vi "EasyFitTransients.vi"(11 "InputData":T3(array[cluster])=[{"JV metrics"=[0.0, 0.004688074, 0.005002861, 0.0053417254, 0.0056762234, 0.0060026976, 0.006369476, 0.0066977106, 0.0070325956, 0.007371202, 0.007696711, 0.008035217, 0.008369455, 0.008697365, 0.0090301, 0.009363418, 0.009698967, 0.010032594, 0.010363362, 0.010703604, 0.01102955, 0.011368416, 0.011698721, 0.012031753, 0.012363813, 0.012696692, 0.013029694, 0.0133624505, 0.013696079, 0.014036833, 0.0143676335, 0.014702026, 0.015034515, 0.015362716, 0.01570068, 0.016029574, 0.016367266, 0.016696516, 0.017030975, 0.01736351, 0.017702773, 0.01802998, 0.018363293, 0.018697608, 0.019032346, 0.019362444, 0.019695722, 0.020032562, 0.0203697], "JV metrics"=[0.69321656, -3.15312e-05, -0.00017485018, -3.621295e-05, 6.4908316e-05, -2.1567195e-05, -2.285478e-05, -7.566182e-05, -0.00020427264, 4.1995507e-05, -0.00015639109, -0.00020229832, -0.00010161646, -0.0001144569, -0.00020186052, -0.00013796492, -0.00014203244, 8.4075975e-05, -2.4384806e-05, -7.140644e-05, 0.00012004285, -7.328456e-06, -0.00010339845, 0.0001509544, 4.349697e-05, 6.881247e-05, -0.0001570559, -3.9619877e-06, -0.00022902519, -4.6681085e-05, -0.0001399173, 7.6152726e-05, -0.0001232961, -0.00024506752, -0.00010704884, -0.00012851319, -0.00014125218, -7.473238e-07, 0.0001521912, -1.1394733e-05, -0.00019358074, 9.507881e-06, 1.6228494e-05, 5.089255e-05, 0.00014946784, 0.00020754292, -0.00022141216, -9.01446e-05, 5.6048953e-05]}]) -> ()   [LabVIEW 2020]
uses:
  <vilib>/Analysis/NI_AALPro.lvlib
panel:
  out "T80 (h)":dbl[](array[numeric])=[nan]
  in  "linear fit: parameter bounds":T1={"slope min"=-inf, "slope max"=inf, "intercept min"=-inf, "intercept max"=inf}
  in  "exponential fit parameter bounds":T2={"amp min"=-inf, "amp max"=inf, "damping min"=-inf, "damping max"=inf, "offset min"=0.0, "offset max"=0.0}
  out "Fitresults":dbl[][](array[numeric])=[[nan, nan, 0.0, nan]]
  out "Cursors":dbl[](array[numeric])=[0.7645161290322581, 5.903225806451613]
  in  "Exit Button":bool
  in  "Fit Button":bool
  in  "Fit function":bool
  out "AgingData":T3(graph)
  # "tau (h) / m (1/h)     A                     c             residue"
  # "from (h):"
  # "exponential\nAexp(dx)+c"
  # "linear\nmt +c"
  # "to (h):"
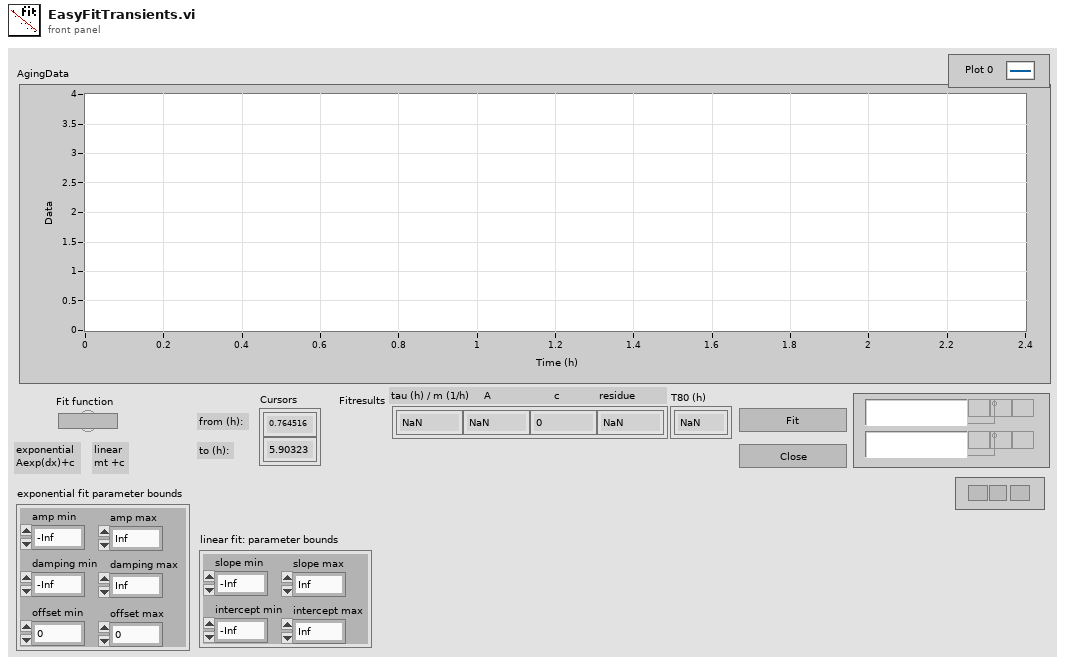
[diagram p1: front panel]
types:
  T1 = cluster{"slope min":dbl, "slope max":dbl, "intercept min":dbl, "intercept max":dbl}
  T2 = cluster{"amp min":dbl, "amp max":dbl, "damping min":dbl, "damping max":dbl, "offset min":dbl, "offset max":dbl}
  T3 = cluster{"JV metrics":sgl[], "JV metrics":sgl[]}[]
  T4 = typedef "LVCursorListTypeDef.ctl" = cluster{"Name":string, "Color":u32, "Style":u8, "Point Style":u8, "Name Visible":bool, "Allow Drag":bool, "Cursor Mode":u32, "Plot":i32, "Index":i32, "Position":cluster{"X":dbl, "Y":dbl}, "X Scale":u32, "Y Scale":u32, "Watch Plots":i32[], "Watch All Plots":bool, "Plot Area":i32, "Label Offset":cluster{"X":dbl, "Y":dbl}}[]
  T5 = cluster{"Name":string, "Color":u32, "Style":u8, "Point Style":u8, "Name Visible":bool, "Allow Drag":bool, "Cursor Mode":u32, "Plot":i32, "Index":i32, "Position":cluster{"X":dbl, "Y":dbl}, "X Scale":u32, "Y Scale":u32, "Watch Plots":i32[], "Watch All Plots":bool, "Plot Area":i32, "Label Offset":cluster{"X":dbl, "Y":dbl}}
  T6 = cluster{"JV metrics":sgl[], "Best Linear Fit":dbl[]}[]
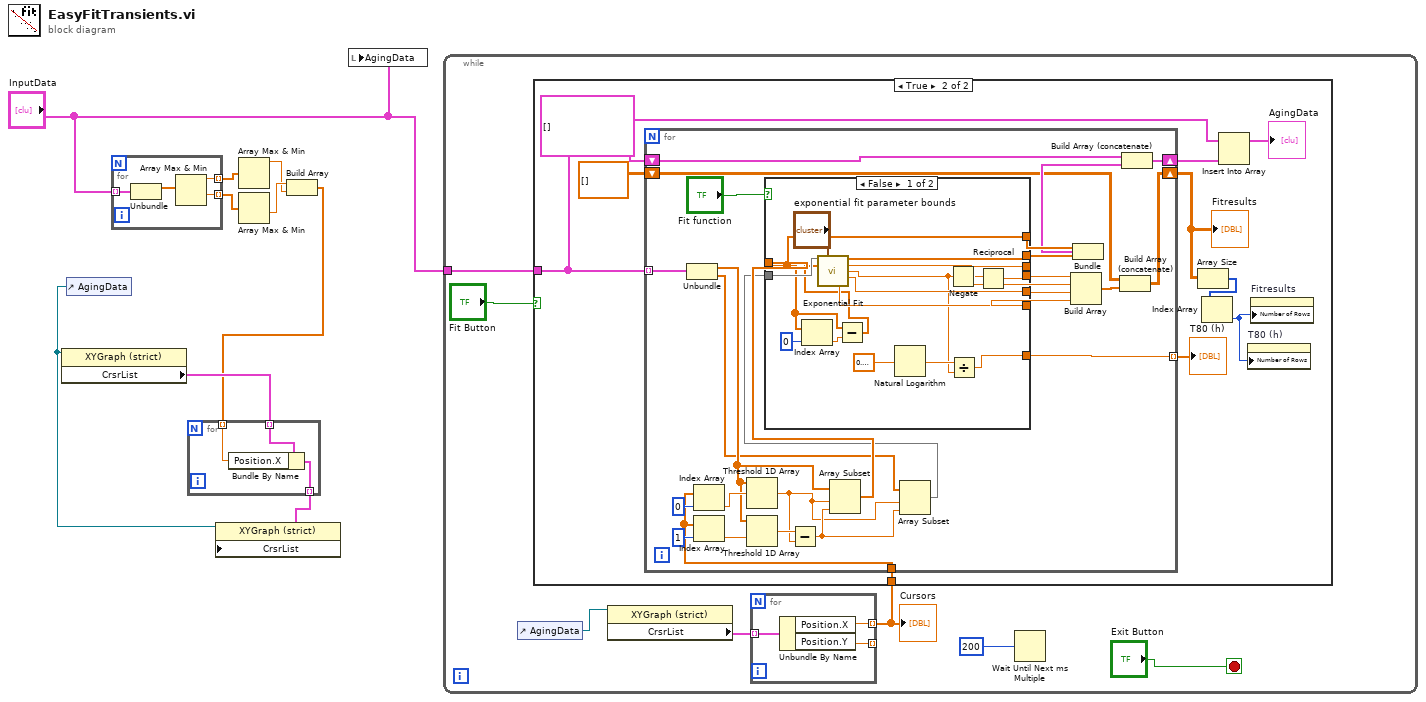
[diagram p0: block diagram]
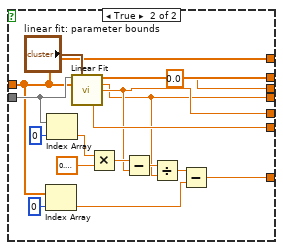
[diagram p3: hidden frame]
diagram:
  n1 = control-ref of="AgingData"() -> (w9:refnum<vi>)
  n2 = property class="XYGraph (strict)"(reference=w9) -> ("CrsrList"=w8:T4)  [unwired: 1 in, 2 out]
  n3 = for {
    tunnel: "InputData" -> [w13] mode=indexing
    tunnel: [w11] -> w6 mode=indexing
    tunnel: [w10] -> w5 mode=indexing
    n4 = Unbundle(w13) -> ("JV metrics"=w12:sgl[])  [unwired: 1 out]
    n5 = Array Max & Min(array=w12) -> (max value=w10:sgl, min value=w11:sgl)  [unwired: 2 out]
  }
  n6 = Array Max & Min(array=w5) -> (max value=w3:sgl)  [unwired: 3 out]
  n7 = Array Max & Min(array=w6) -> (min value=w4:sgl)  [unwired: 3 out]
  n8 = Build Array(w4, w3) -> (w2:sgl[])
  n9 = for {
    tunnel: w8 -> [w16] mode=indexing
    tunnel: [w15] -> w7 mode=indexing
    tunnel: w2 -> [w14] mode=indexing
    n10 = Bundle By Name(cluster=w16, "Position.X"=w14) -> (w15:T5)
  }
  n11 = property class="XYGraph (strict)"(reference=w9, "CrsrList"=w7) -> ()  [unwired: 1 in, 2 out]
  n12 = local write "AgingData"("InputData") -> ()
  n13 = while {
    tunnel: "InputData" -> [w23]
    stop <- "Exit Button" stop-if-true
    n14 = control-ref of="AgingData"() -> (w18:refnum<vi>)
    n15 = property class="XYGraph (strict)"(reference=w18) -> ("CrsrList"=w19:T4)  [unwired: 1 in, 2 out]
    n16 = for {
      tunnel: w19 -> [w26] mode=indexing
      tunnel: [w25] -> w17 mode=indexing
      tunnel: [w24] -> _ mode=indexing
      n17 = Unbundle By Name(w26) -> ("Position.X"=w25:dbl, "Position.Y"=w24:dbl)
    }
    "Cursors" <- w17
    n18 = case shown="True" "Fit Button" {
      tunnel: w23 -> [_ w35]
      tunnel: w17 -> [_ w29]
      frame False {
      }
      frame True {
        n19 = for {
          tunnel: w35 -> [w63] mode=indexing
          shift-right: [w58] -> w34
          shift-left: T6 [] -> [w57]
          shift-right: [w51] -> w30
          shift-left: dbl[][] [] -> [w50]
          tunnel: w29 -> [w45]
          tunnel: [w37] -> w28 mode=indexing
          n20 = Unbundle(w63) -> ("JV metrics"=w43:sgl[], "JV metrics"=w39:sgl[])
          n21 = Index Array(array=w45, index=0) -> (element=w48:dbl)
          n22 = Index Array(array=w45, index=1) -> (element=w47:dbl)
          n23 = Threshold 1D Array(2:w48, 3:w43) -> (0:w40:sgl)  [unwired: 1 in]
          n24 = Threshold 1D Array(2:w47, 3:w43) -> (0:w44:sgl)  [unwired: 1 in]
          n25 = Subtract(x=w44, y=w40) -> (x-y=w41:sgl)
          n26 = Array Subset(array=w43, index=w40, length=w41) -> (w42:sgl[])
          n27 = Array Subset(array=w39, index=w40, length=w41) -> (w38:sgl[])
          n28 = case shown="False" "Fit function" {
            tunnel: w38 -> [w79 w88]
            tunnel: w42 -> [w70 w86]
            tunnel: [w78 w96] -> w60
            tunnel: [w70 w86] -> w61
            tunnel: [w72 w82] -> w56
            tunnel: [w77 0.0 ("offset")] -> w55
            tunnel: [w75 w95] -> w54
            tunnel: [w76 w83] -> w53
            tunnel: [w64 w80] -> w37
            frame False {
              n29 = Index Array(array=w70, index=0) -> (element=w69:sgl)
              n30 = Subtract(x=w70, y=w69) -> (x-y=w68:sgl[])
              n31 = call <vilib>:"Exponential Fit.vi"("Y"=w79, "X"=w68, "parameter bounds"="exponential fit parameter bounds") -> ("Best Exponential Fit"=w78:dbl[], "amplitude"=w77:dbl, "damping"=w65:dbl, "offset"=w76:dbl, "residue"=w75:dbl)  [unwired: 7 in, 1 out]
              n32 = Natural Logarithm(1:sgl 0.8 ("y")) -> (0:w66:sgl)
              n33 = Negate(x=w65) -> (-x=w73:dbl)
              n34 = Divide(x=w66, y=w65) -> (x/y=w64:dbl)
              n35 = Reciprocal(x=w73) -> (1/x=w72:dbl)
            }
            frame True {
              n36 = Index Array(array=w86, index=0) -> (element=w81:sgl)
              n37 = Index Array(array=w88, index=0) -> (element=w85:sgl)
              n38 = call <vilib>:"Linear Fit.vi"("Y"=w88, "X"=w86, "parameter bounds"="linear fit: parameter bounds") -> ("Best Linear Fit"=w96:dbl[], "slope"=w82:dbl, "intercept"=w83:dbl, "residue"=w95:dbl)  [unwired: 8 in, 1 out]
              n39 = Multiply(x=w85, y=sgl 0.8) -> (x*y=w92:sgl)
              n40 = Subtract(x=w92, y=w83) -> (x-y=w91:dbl)
              n41 = Divide(x=w91, y=w82) -> (x/y=w90:dbl)
              n42 = Subtract(x=w90, y=w81) -> (x-y=w80:dbl)
            }
          }
          n43 = Build Array(w56, w55, w53, w54) -> (w52:dbl[])
          n44 = Bundle(w61, "Best Linear Fit"=w60) -> (w59:cluster{sgl[], "Best Linear Fit":dbl[]})  [unwired: 1 in]
          n45 = Build Array (concatenate)(w50, w52) -> (w51:dbl[][])
          n46 = Build Array (concatenate)(w57, w59) -> (w58:T6)
        }
        "Fitresults" <- w30
        "T80 (h)" <- w28
        n47 = Array Size(array=w30) -> (size(s)=w31:i32[])
        n48 = Index Array(array=w31) -> (element=w27:i32)  [unwired: 1 in]
        n49 = Insert Into Array(array=w35, new element=w34) -> (→"AgingData":T3)  [unwired: 1 in]
        n50 = property on="T80 (h)" class="Arr (strict)"("Number of Rows"=w27) -> ()  [unwired: 2 in, 2 out]
        n51 = property on="Fitresults" class="Arr (strict)"("Number of Rows"=w27) -> ()  [unwired: 2 in, 2 out]
      }
    }
    n52 = Wait Until Next ms Multiple(millisecond multiple=u32 200) -> ()  [unwired: 1 out]
  }
